vi "Example.vi"() -> ()   [LabVIEW 2015]
uses:
  <vilib>/Platform/TimedLoop/XDataNode/wakeup.ctl
  <vilib>/Platform/TimedLoop/XDataNode/XDNodeRunTimeDep.lvlib
  <vilib>/Platform/TimedLoop/XDataNode/nitl_modes.ctl
  <vilib>/Platform/TimedLoop/XDataNode/timing_clust.ctl
  <vilib>/Platform/TimedLoop/XDataNode/XDataNode.xnode
  <vilib>/NI/Engine Simulation Toolkit (EST)/APU/APU.lvlib
  <vilib>/rvi/DataTransferAndStorage/Container/XNode/niFpgaContainer.xnode
  <vilib>/rvi/interface/RandomDataEmulation/nirviRandomDataFpgaReadWriteTemplate.vi
  <vilib>/NI/Engine Simulation Toolkit (EST)/Directional Speed/Directional Speed.lvlib
  <vilib>/NI/Engine Simulation Toolkit (EST)/Digital Pattern Generation/Digital Pattern Generation.lvlib
  <vilib>/NI/Engine Simulation Toolkit (EST)/Analog Replay/Analog Replay.lvlib
  <vilib>/NI/FPGA Addon IP/Speciality IO/Speciality FPGA IO.lvlib
  <vilib>/NI/Engine Simulation Toolkit (EST)/Knock Sensor/Knock Sensor.lvlib
  <vilib>/NI/Engine Simulation Toolkit (EST)/ECU Event/Timing/ECU Event Timing.lvlib
  <vilib>/NI/Engine Simulation Toolkit (EST)/ECU Event/Timing/Measure Events (Non-40MHz).vi
  <vilib>/NI/Engine Simulation Toolkit (EST)/ECU Event/Timing/Capture Settings.ctl
  <vilib>/NI/Engine Simulation Toolkit (EST)/APU/Shared Settings.ctl
  <vilib>/NI/Engine Simulation Toolkit (EST)/Version Token.ctl
  <vilib>/NI/Engine Simulation Toolkit (EST)/Engine Simulation Toolkit.lvlib
  <vilib>/NI/Engine Simulation Toolkit (EST)/APU/Settings.ctl
  <vilib>/NI/Engine Simulation Toolkit (EST)/APU/Input.ctl
  <vilib>/NI/Engine Simulation Toolkit (EST)/APU/Output.ctl
  <vilib>/NI/Engine Simulation Toolkit (EST)/Directional Speed/Load Input.ctl
  <vilib>/NI/Engine Simulation Toolkit (EST)/Digital Pattern Generation/Load Input.ctl
  <vilib>/NI/Engine Simulation Toolkit (EST)/Analog Replay/Load Input.ctl
  <vilib>/NI/FPGA Addon IP/Speciality IO/Types/PWM.Measure.Analog.Settings.ctl
  <vilib>/NI/FPGA Addon IP/Speciality IO/Types/PWM.Measure.Analog.Measurement.ctl
  <vilib>/NI/Engine Simulation Toolkit (EST)/Knock Sensor/Cylinder Settings.ctl
  <vilib>/NI/Engine Simulation Toolkit (EST)/Knock Sensor/Cylinder Input.ctl
  <vilib>/NI/Engine Simulation Toolkit (EST)/Knock Sensor/Generate Settings.ctl
  <vilib>/NI/Engine Simulation Toolkit (EST)/Knock Sensor/Generate Input.ctl
  <vilib>/NI/FPGA Addon IP/Speciality IO/Types/Sine.Generate.Settings.ctl
  <vilib>/NI/Engine Simulation Toolkit (EST)/Analog Replay/Input.ctl
  <vilib>/NI/Engine Simulation Toolkit (EST)/Analog Replay/Settings.ctl
  <vilib>/NI/Engine Simulation Toolkit (EST)/Directional Speed/Input.ctl
  <vilib>/NI/Engine Simulation Toolkit (EST)/Directional Speed/Settings.ctl
  <vilib>/NI/Engine Simulation Toolkit (EST)/Digital Pattern Generation/Input.ctl
  <vilib>/NI/Engine Simulation Toolkit (EST)/Digital Pattern Generation/Settings.ctl
  <vilib>/NI/FPGA Addon IP/Speciality IO/Types/PWM.Generate.Digital.Settings.ctl
  <vilib>/NI/FPGA Addon IP/Speciality IO/Types/WSS.Generate.Digital.Settings.ctl
  <vilib>/NI/Engine Simulation Toolkit (EST)/ECU Event/Timing/Measure Settings.ctl
  <vilib>/NI/Engine Simulation Toolkit (EST)/ECU Event/Timing/Measure Output.ctl
  <vilib>/NI/Engine Simulation Toolkit (EST)/ECU Event/Timing/Capture Output.ctl
  <vilib>/NI/FPGA Addon IP/Speciality IO/Types/PWM.Measure.Digital.Settings.ctl
  <vilib>/NI/FPGA Addon IP/Speciality IO/Types/PWM.Measure.Digital.Measurement.ctl
panel:
  out "Switch State":bool
  out "Relay State":bool
  out "PWM IN 2.Measure":T1
  in  "PWM IN 2.Settings":T2={"ACTIVE EDGE"=TRUE, "TIMEOUT"=40000000}
  out "PWM IN 1.Measure":T1
  in  "PWM IN 1.Settings":T2={"ACTIVE EDGE"=TRUE, "TIMEOUT"=40000000}
  out "Key State":bool
  out "capture.Cyl Inj 3.Event 4":T3
  out "capture.Cyl Inj 3.Event 3":T3
  out "capture.Cyl Inj 3.Event 2":T3
  out "capture.Cyl Inj 3.Event 1":T3
  out "status.Cyl Inj 3":T4
  in  "settings.Cyl Inj 3":T5
  out "capture.Cyl Inj 2.Event 4":T3
  out "capture.Cyl Inj 2.Event 3":T3
  out "capture.Cyl Inj 2.Event 2":T3
  out "capture.Cyl Inj 2.Event 1":T3
  out "status.Cyl Inj 2":T4
  in  "settings.Cyl Inj 2":T5
  out "capture.Cyl Inj 1.Event 4":T3
  out "capture.Cyl Inj 1.Event 3":T3
  out "capture.Cyl Inj 1.Event 2":T3
  out "capture.Cyl Inj 1.Event 1":T3
  out "status.Cyl Inj 1":T4
  in  "settings.Cyl Inj 1":T5
  out "Test.Monitor":bool[](array[boolean])
  out "Mod5.Monitor":bool[](array[boolean])
  in  "Rear Driver WS.Settings":T6={"ACTIVE EDGE"=TRUE, "ACTIVE TICKS"=0, "INACTIVE TICKS"=0, "DATA"=0, "SENSOR TYPE"=0}
  in  "Read Passenger WS.Settings":T6={"ACTIVE EDGE"=TRUE, "ACTIVE TICKS"=0, "INACTIVE TICKS"=0, "DATA"=0, "SENSOR TYPE"=0}
  in  "Front Passenger WS.Settings":T6={"ACTIVE EDGE"=TRUE, "ACTIVE TICKS"=0, "INACTIVE TICKS"=0, "DATA"=0, "SENSOR TYPE"=0}
  in  "Front Driver WS.Settings":T6={"ACTIVE EDGE"=TRUE, "ACTIVE TICKS"=0, "INACTIVE TICKS"=0, "DATA"=0, "SENSOR TYPE"=0}
  out "Mod3.Monitor":bool[](array[boolean])
  in  "Switch":bool
  in  "PWM Out 2.Settings":T7={"ACTIVE EDGE"=TRUE, "ACTIVE TICKS"=0, "INACTIVE TICKS"=0}
  in  "PWM Out 1.Settings":T7={"ACTIVE EDGE"=TRUE, "ACTIVE TICKS"=0, "INACTIVE TICKS"=0}
  in  "Key":bool
  in  "input.Intake CAM 1":T8
  in  "settings.Intake CAM 1":T9
  in  "input.Exhaust CAM 1":T8
  in  "settings.Exhaust CAM 1":T9
  in  "input.Crank_Temp":T8
  in  "settings.Crank_Temp":T9
  in  "input.Crank":T10
  in  "settings.Crank":T11
  out "Mod4.Monitor":fxp<+/-,32,8>[](array[numeric])
  in  "input.VR Sensor4":T12
  in  "settings.VR Sensor4":T13
  in  "input.VR Sensor3":T12
  in  "settings.VR Sensor3":T13
  in  "input.VR Sensor2":T12
  in  "settings.VR Sensor2":T13
  in  "input.VR Sensor1":T12
  in  "settings.VR Sensor1":T13
  in  "Simple Knock 2.Settings":T14={"AMP"=0.0, "OFFSET"=0.0, "PERIODS/TICKS"=2.4999957531690598e-05}
  in  "Simple Knock 1.Settings":T14={"AMP"=0.0, "OFFSET"=0.0, "PERIODS/TICKS"=2.4999957531690598e-05}
  in  "Power Supply Setpoint":fxp<+/-,32,8> format="%#_27g"
  in  "input.Knock2":T15
  in  "settings.Knock2":T16
  in  "input.Knock2.Cylinder 6":T17={"probability compare"=65535, "high freq scaler"=0.0, "trigger position"=0}
  in  "settings.Knock2.Cylinder 6":T18
  in  "input.Knock2.Cylinder 5":T17={"probability compare"=65535, "high freq scaler"=0.0, "trigger position"=0}
  in  "settings.Knock2.Cylinder 5":T18
  in  "input.Knock2.Cylinder 4":T17={"probability compare"=65535, "high freq scaler"=0.0, "trigger position"=0}
  in  "settings.Knock2.Cylinder 4":T18
  in  "input.Knock2.Cylinder 3":T17={"probability compare"=65535, "high freq scaler"=0.0, "trigger position"=0}
  in  "settings.Knock2.Cylinder 3":T18
  in  "input.Knock2.Cylinder 2":T17={"probability compare"=65535, "high freq scaler"=0.0, "trigger position"=0}
  in  "settings.Knock2.Cylinder 2":T18
  in  "input.Knock2.Cylinder 1":T17={"probability compare"=65535, "high freq scaler"=0.0, "trigger position"=0}
  in  "settings.Knock2.Cylinder 1":T18
  in  "input.Knock1":T15
  in  "settings.Knock1":T16
  in  "input.Knock1.Cylinder 6":T17={"probability compare"=65535, "high freq scaler"=0.0, "trigger position"=0}
  in  "settings.Knock1.Cylinder 6":T18
  in  "input.Knock1.Cylinder 5":T17={"probability compare"=65535, "high freq scaler"=0.0, "trigger position"=0}
  in  "settings.Knock1.Cylinder 5":T18
  in  "input.Knock1.Cylinder 4":T17={"probability compare"=65535, "high freq scaler"=0.0, "trigger position"=0}
  in  "settings.Knock1.Cylinder 4":T18
  in  "input.Knock1.Cylinder 3":T17={"probability compare"=65535, "high freq scaler"=0.0, "trigger position"=0}
  in  "settings.Knock1.Cylinder 3":T18
  in  "input.Knock1.Cylinder 2":T17={"probability compare"=65535, "high freq scaler"=0.0, "trigger position"=0}
  in  "settings.Knock1.Cylinder 2":T18
  in  "input.Knock1.Cylinder 1":T17={"probability compare"=65535, "high freq scaler"=0.0, "trigger position"=0}
  in  "settings.Knock1.Cylinder 1":T18
  in  "Dyno Setpoint":fxp<+/-,32,8> format="%#_27g"
  out "Temp4":fxp<+/-,32,8> format="%#_27g"
  out "Temp3":fxp<+/-,32,8> format="%#_27g"
  out "Temp2":fxp<+/-,32,8> format="%#_27g"
  out "Temp1":fxp<+/-,32,8> format="%#_27g"
  out "Pressure2":fxp<+/-,32,8> format="%#_27g"
  out "Pressure1":fxp<+/-,32,8> format="%#_27g"
  out "Injector4.Measure":T19
  in  "Injector4.Settings":T20={"ACTIVE EDGE"=TRUE, "TIMEOUT"=40000000, "THRESHOLD"=50.0}
  out "Injector3.Measure":T19
  in  "Injector3.Settings":T20={"ACTIVE EDGE"=TRUE, "TIMEOUT"=40000000, "THRESHOLD"=50.0}
  out "Injector2.Measure":T19
  in  "Injector2.Settings":T20={"ACTIVE EDGE"=TRUE, "TIMEOUT"=40000000, "THRESHOLD"=50.0}
  out "Injector1.Measure":T19
  in  "Injector1.Settings":T20={"ACTIVE EDGE"=TRUE, "TIMEOUT"=40000000, "THRESHOLD"=50.0}
  out "Mod2.Monitor":fxp<+/-,24,5>[](array[numeric])
  in  "load input.VR Sensor4":T21={"Data"=[0, 0, 0, 0, 0, 0, 0, 0, 0, 0, 0, 0, 0, 0, 0, 0], "LoadOffset"=0, "Done"=FALSE}
  in  "load input.VR Sensor3":T21={"Data"=[0, 0, 0, 0, 0, 0, 0, 0, 0, 0, 0, 0, 0, 0, 0, 0], "LoadOffset"=0, "Done"=FALSE}
  in  "load input.VR Sensor2":T21={"Data"=[0, 0, 0, 0, 0, 0, 0, 0, 0, 0, 0, 0, 0, 0, 0, 0], "LoadOffset"=0, "Done"=FALSE}
  in  "load input.VR Sensor1":T21={"Data"=[0, 0, 0, 0, 0, 0, 0, 0, 0, 0, 0, 0, 0, 0, 0, 0], "LoadOffset"=0, "Done"=FALSE}
  in  "load input.Intake CAM 1":T22
  in  "load input.Exhaust CAM 1":T22
  in  "load input.Crank_Temp":T22
  in  "load input.Crank":T23
  in  "Analog Input Loop Timer (uSec)":u32
  out "output.apu 1":T24 caption="output"
  in  "input.apu 1":T25={"desired speed"=0.0, "reset"=TRUE} caption="input"
  in  "settings.apu 1":T26 caption="settings"
  in  "est.version":T27
  in  "shared settings.apu 1":T28 {"start" format="%#.15g"}
  in  "go.apu 1":bool
  in  "Digital Loop Timer (uSec)":u32
  in  "Analog Output Loop Timer (uSec)":u32
  in  "DMA.Enable":bool
  in  "DMA.MinimumSamples":u32 caption="DMA Loop Timer (uSec)"
  out "DMA.Timeout":bool
  in  "DMA.Timeout.Reset":bool
  in  "DMA Loop Timer (uSec)":u32
types:
  T1 = typedef "Speciality FPGA IO.lvlib/PWM.Measure.Digital.Measurement.ctl" = cluster{"ACTIVE TICKS":u32, "INACTIVE TICKS":u32, "ACQ TICKS":u32}
  T2 = typedef "Speciality FPGA IO.lvlib/PWM.Measure.Digital.Settings.ctl" = cluster{"ACTIVE EDGE":bool, "TIMEOUT":u32}
  T3 = typedef "Engine Simulation Toolkit.lvlib/ECU Event Timing.lvlib/Capture Output.ctl" = cluster{"Start":u16, "End":u16, "Duration (tics)":fxp<+,18,18>, "Event present":bool}
  T4 = typedef "Engine Simulation Toolkit.lvlib/ECU Event Timing.lvlib/Measure Output.ctl" = cluster{"stuck active":bool, "window all active":bool, "window orphan start":bool, "window orphan end":bool}
  T5 = typedef "Engine Simulation Toolkit.lvlib/ECU Event Timing.lvlib/Measure Settings.ctl" = cluster{"max":u16, "min":u16, "active high":bool, "wrap":bool}
  T6 = typedef "Speciality FPGA IO.lvlib/WSS.Generate.Digital.Settings.ctl" = cluster{"ACTIVE EDGE":bool, "ACTIVE TICKS":u32, "INACTIVE TICKS":u32, "DATA":u8, "SENSOR TYPE":u8}
  T7 = typedef "Speciality FPGA IO.lvlib/PWM.Generate.Digital.Settings.ctl" = cluster{"ACTIVE EDGE":bool, "ACTIVE TICKS":u32, "INACTIVE TICKS":u32}
  T8 = typedef "Engine Simulation Toolkit.lvlib/Digital Pattern Generation.lvlib/Settings.ctl" = cluster{"edge 1":u16, "edge 2":u16, "cycle angle":bool, "enabled":bool, "first falling":bool, "fault":bool, "fault wrap":bool, "fault value":bool, "fault count":fxp<+,4,4>, "use fault count":bool}
  T9 = typedef "Engine Simulation Toolkit.lvlib/Digital Pattern Generation.lvlib/Input.ctl" = cluster{"Offset":i16}
  T10 = typedef "Engine Simulation Toolkit.lvlib/Directional Speed.lvlib/Settings.ctl" = cluster{"Upper Value":u16, "Lower Value":u16, "Upper Index":fxp<+,10,10>, "Lower Index":fxp<+,10,10>, "Enabled":bool}
  T11 = typedef "Engine Simulation Toolkit.lvlib/Directional Speed.lvlib/Input.ctl" = cluster{"td (tics)":u16, "tf (tics)":u16, "tr (tics)":u16}
  T12 = typedef "Engine Simulation Toolkit.lvlib/Analog Replay.lvlib/Settings.ctl" = cluster{"ReverseNegate":bool, "CycleAngle":bool, "SpeedThreshold":fxp<+/-,23,2>, "AOBelowThreshold":i16}
  T13 = typedef "Engine Simulation Toolkit.lvlib/Analog Replay.lvlib/Input.ctl" = cluster{"Offset":i16, "VScaleSlope":fxp<+,18,6>, "VScaleIntercept":fxp<+/-,18,3>}
  T14 = typedef "Speciality FPGA IO.lvlib/Sine.Generate.Settings.ctl" = cluster{"AMP":fxp<+/-,32,8>, "OFFSET":fxp<+/-,32,8>, "PERIODS/TICKS":fxp<+,32,0>}
  T15 = typedef "Engine Simulation Toolkit.lvlib/Knock Sensor.lvlib/Generate Input.ctl" = cluster{"low freq scaler":fxp<+,10,0>}
  T16 = typedef "Engine Simulation Toolkit.lvlib/Knock Sensor.lvlib/Generate Settings.ctl" = cluster{"low freq (periods/tick)":fxp<+,32,0>, "high freq (periods/tick)":fxp<+,32,0>, "duration (1.25MHz tics)":fxp<+,18,18>, "low freq speed slope":fxp<+,16,-3>, "low freq speed intercept":fxp<+,10,-10>, "low freq by speed":bool}
  T17 = typedef "Engine Simulation Toolkit.lvlib/Knock Sensor.lvlib/Cylinder Input.ctl" = cluster{"probability compare":u16, "high freq scaler":fxp<+,10,0>, "trigger position":u16}
  T18 = typedef "Engine Simulation Toolkit.lvlib/Knock Sensor.lvlib/Cylinder Settings.ctl" = cluster{"seed":u16, "reset":bool}
  T19 = typedef "Speciality FPGA IO.lvlib/PWM.Measure.Analog.Measurement.ctl" = cluster{"ACTIVE TICKS":u32, "INACTIVE TICKS":u32, "ACQ TICKS":u32, "ACTIVE VOLTAGE":fxp<+/-,32,8>, "INACTIVE VOLTAGE":fxp<+/-,32,8>}
  T20 = typedef "Speciality FPGA IO.lvlib/PWM.Measure.Analog.Settings.ctl" = cluster{"ACTIVE EDGE":bool, "TIMEOUT":u32, "THRESHOLD":fxp<+/-,32,8>}
  T21 = typedef "Engine Simulation Toolkit.lvlib/Analog Replay.lvlib/Load Input.ctl" = cluster{"Data":i16[], "LoadOffset":u16, "Done":bool}
  T22 = typedef "Engine Simulation Toolkit.lvlib/Digital Pattern Generation.lvlib/Load Input.ctl" = cluster{"address":fxp<+,11,11>, "done":bool, "angle":u16}
  T23 = typedef "Engine Simulation Toolkit.lvlib/Directional Speed.lvlib/Load Input.ctl" = cluster{"address":fxp<+,10,10>, "done":bool, "angle":u16}
  T24 = typedef "Engine Simulation Toolkit.lvlib/APU.lvlib/Output.ctl" = cluster{"crank":u16, "cycle":u16, "actual speed":fxp<+/-,23,2>}
  T25 = typedef "Engine Simulation Toolkit.lvlib/APU.lvlib/Input.ctl" = cluster{"desired speed":fxp<+/-,23,2>, "reset":bool}
  T26 = typedef "Engine Simulation Toolkit.lvlib/APU.lvlib/Settings.ctl" = cluster{"acceleration":fxp<+,18,-20>, "enable accel":bool}
  T27 = typedef "Engine Simulation Toolkit.lvlib/Version Token.ctl" = cluster{"1.3.0":bool}
  T28 = typedef "Engine Simulation Toolkit.lvlib/APU.lvlib/Shared Settings.ctl" = cluster{"start":fxp<+,17,17>, "stuck limit":fxp<+,18,18>}
  T29 = typedef "XDNodeRunTimeDep.lvlib/timing_clust.ctl" = cluster{"Expected End [f-1]":u64, "Actual End [f-1]":u64, "Finished Late? [f-1]":bool, "Expected End [i-1]":u64, "Actual End [i-1]":u64, "Finished Late? [i-1]":bool, "Expected Start [i]":u64, "Actual Start [i]":u64, "Expected Start [f]":u64, "Actual Start [f]":u64, "Source Name":string, "Structure Name":string, "Period":i64, "Deadline":i64, "Offset":i64, "Start":i64, "Priority":i32, "Timeout":i32, "Mode":T30, "Wakeup Reason":T31, "Error":errorcluster, "Source Type":string, "Secondary Source Type":string, "Global End Time":u64, "Global Start Time":u64, "Frame Duration":u64, "Iteration Duration":u64, "Assigned CPU":i32, "I/O Scan Engine Mode":u32}
  T30 = typedef "XDNodeRunTimeDep.lvlib/nitl_modes.ctl" = enum32{"No Change", "Process missed periods, maintain original phase", "Discard missed periods, maintain original phase", "Process missed periods, ignore original phase", "Discard missed periods, ignore original phase"}
  T31 = typedef "XDNodeRunTimeDep.lvlib/wakeup.ctl" = enum32{"Normal", "Aborted", "Asynchronous wakeup", "Timing source error", "Timed loop error", "Timeout"}
  T32 = typedef "Engine Simulation Toolkit.lvlib/ECU Event Timing.lvlib/Capture Settings.ctl" = u8
  T33 = cluster{"DI 0":refnum<k21>, "DI 1":refnum<k21>, "DI 2":refnum<k21>, "DI 3":refnum<k21>, "DI 4":refnum<k21>, "DI 5":refnum<k21>, "DI 6":refnum<k21>, "DI 7":refnum<k21>}
  T34 = cluster{"DO 0":refnum<k21>, "DO 1":refnum<k21>, "DO 2":refnum<k21>, "DO 3":refnum<k21>, "DO 4":refnum<k21>, "DO 5":refnum<k21>, "DO 6":refnum<k21>, "DO 7":refnum<k21>}
  T35 = cluster{"AO 0":refnum<k21>, "AO 1":refnum<k21>, "AO 2":refnum<k21>, "AO 3":refnum<k21>, "AO 4":refnum<k21>, "AO 5":refnum<k21>, "AO 6":refnum<k21>, "AO 7":refnum<k21>, "AO 8":refnum<k21>, "AO 9":refnum<k21>, "AO 10":refnum<k21>, "AO 11":refnum<k21>, "AO 12":refnum<k21>, "AO 13":refnum<k21>, "AO 14":refnum<k21>, "AO 15":refnum<k21>}
  T36 = cluster{"AI 0":refnum<k21>, "AI 1":refnum<k21>, "AI 2":refnum<k21>, "AI 3":refnum<k21>, "AI 4":refnum<k21>, "AI 5":refnum<k21>, "AI 6":refnum<k21>, "AI 7":refnum<k21>, "AI 8":refnum<k21>, "AI 9":refnum<k21>, "AI 10":refnum<k21>, "AI 11":refnum<k21>, "AI 12":refnum<k21>, "AI 13":refnum<k21>, "AI 14":refnum<k21>, "AI 15":refnum<k21>}
  T37 = typedef "Engine Simulation Toolkit.lvlib/APU.lvlib/Register Bus.ctl" = cluster{"Speed":refnum<k21>, "Crank Angle":refnum<k21>, "Cycle Angle":refnum<k21>, "Crank Count":refnum<k21>, "Cycle Count":refnum<k21>, "1.25 MHz Counter":refnum<k21>, "Crank Rollover":refnum<k21>, "Cycle Rollover":refnum<k21>, "shared settings":T28}
  T38 = typedef "Engine Simulation Toolkit.lvlib/Directional Speed.lvlib/Load Data.ctl" = cluster{"max address":fxp<+,10,10>, "Memory":refnum<k21>}
  T39 = typedef "Engine Simulation Toolkit.lvlib/Digital Pattern Generation.lvlib/Load Data.ctl" = cluster{"max address":fxp<+,11,11>, "memory":refnum<k21>}
  T40 = typedef "Engine Simulation Toolkit.lvlib/Knock Sensor.lvlib/Triggered Cylinder Data.ctl" = cluster{"trigger knock":bool, "high freq scaler":fxp<+,10,0>}
  T41 = typedef "Engine Simulation Toolkit.lvlib/ECU Event Timing.lvlib/Measured Data.ctl" = cluster{"start":u16, "end":u16, "duration (tics)":fxp<+,18,18>, "window end":bool, "window begin":bool, "pulse end":bool, "pulse #":u8}
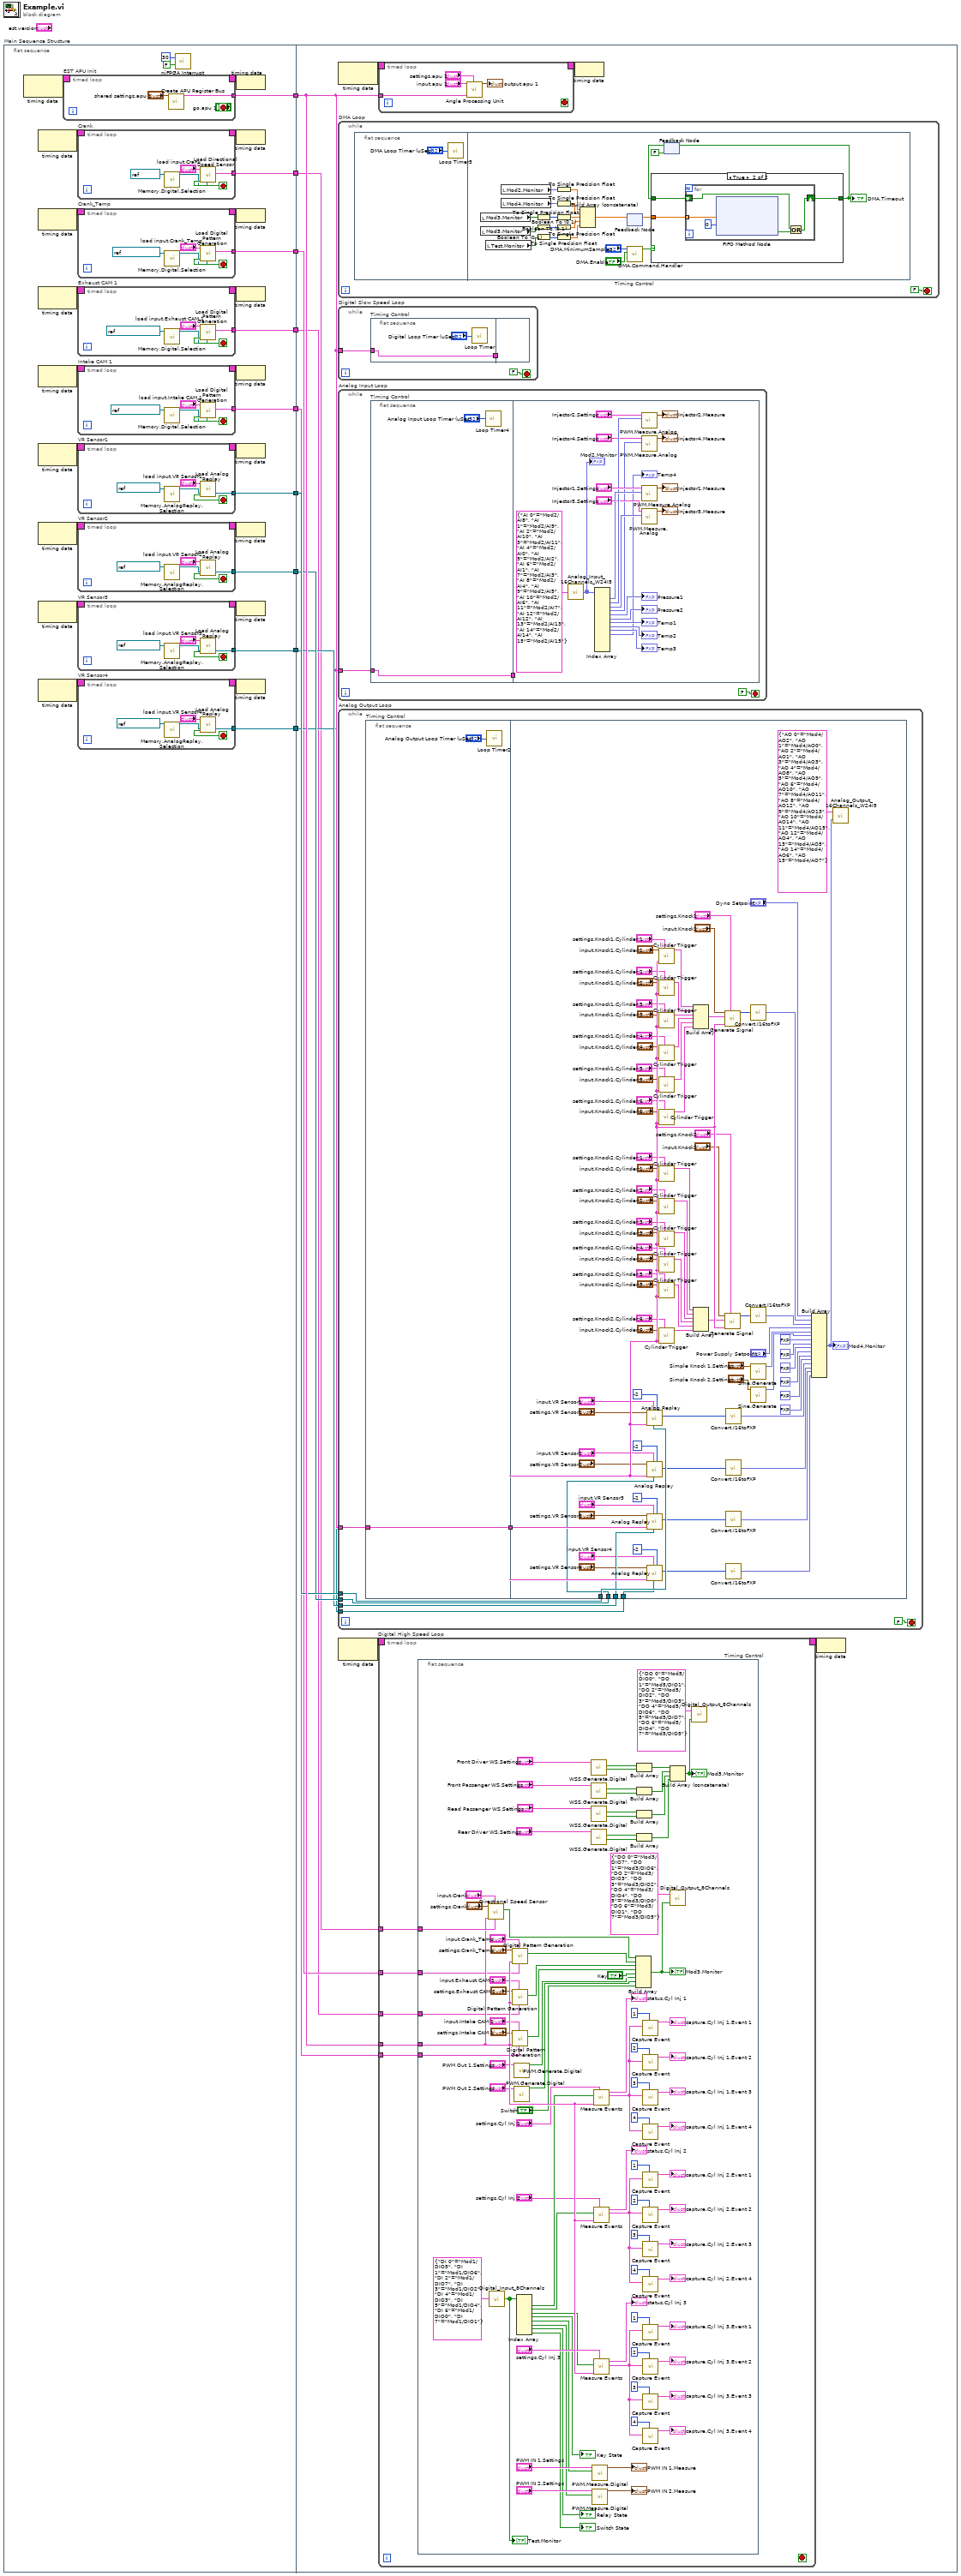
[diagram p0: block diagram]
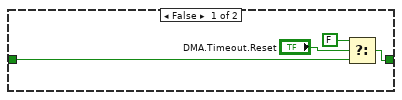
[diagram p2: hidden frame]
diagram:
  n1 = flat-sequence "Main Sequence Structure" {
    tunnel: [w34] -> w9
    tunnel: [w17] -> w8
    tunnel: [w16] -> w7
    tunnel: [w15] -> w6
    tunnel: [w14] -> w5
    tunnel: [w13] -> w4
    tunnel: [w12] -> w3
    tunnel: [w11] -> w2
    tunnel: [w10] -> w1
    tunnel: w9 -> [w122]
    tunnel: w8 -> [w121]
    tunnel: w7 -> [w120]
    tunnel: w6 -> [w119]
    tunnel: w5 -> [w118]
    tunnel: w4 -> [w117]
    tunnel: w3 -> [w116]
    tunnel: w2 -> [w115]
    tunnel: w1 -> [w114]
    frame #0 {
      n2 = node-c288() -> (w36:T29)  [unwired: 1 in]
      n3 = node-c288() -> (w33:T29)  [unwired: 1 in]
      n4 = node-c288() -> (w31:T29)  [unwired: 1 in]
      n5 = node-c288() -> (w29:T29)  [unwired: 1 in]
      n6 = node-c288() -> (w27:T29)  [unwired: 1 in]
      n7 = node-c288() -> (w25:T29)  [unwired: 1 in]
      n8 = node-c288() -> (w23:T29)  [unwired: 1 in]
      n9 = node-c288() -> (w21:T29)  [unwired: 1 in]
      n10 = node-c288() -> (w19:T29)  [unwired: 1 in]
      n11 = timed-loop "EST APU Init" {
        timing: w36 -> [_]
        timing-out: [_] -> w35
        tunnel: [w107] -> w34
        stop <- "go.apu 1" stop-if-true
        n12 = call <vilib>:"Create APU Register Bus.vi"("shared settings.<user name>"="shared settings.apu 1") -> ("register bus"=w107:T37)  [unwired: 10 in]
      }
      n13 = timed-loop "Crank" {
        timing: w33 -> [_]
        timing-out: [_] -> w32
        tunnel: [w98] -> w13
        stop <- w101 stop-if-true
        n14 = call "Memory.Digital.Selection.vi"("memory"=refnum<k21> "Crank") -> ("memory"=w99:refnum<k21>)  [unwired: 10 in]
        n15 = call <vilib>:"Load Directional Speed Sensor.vi"("Memory In"=w99, "load input.<user name>"="load input.Crank") -> ("done"=w101:bool, "load data"=w98:T38)  [unwired: 8 in]
      }
      n16 = timed-loop "Crank_Temp" {
        timing: w31 -> [_]
        timing-out: [_] -> w30
        tunnel: [w89] -> w12
        stop <- w92 stop-if-true
        n17 = call "Memory.Digital.Selection.vi"("memory"=refnum<k21> "Crank_Temp") -> ("memory"=w90:refnum<k21>)  [unwired: 10 in]
        n18 = call <vilib>:"Load Digital Pattern Generation.vi"("memory"=w90, "load input.<user name>"="load input.Crank_Temp") -> ("done"=w92:bool, "load data"=w89:T39)  [unwired: 8 in]
      }
      n19 = timed-loop "Exhaust CAM 1" {
        timing: w29 -> [_]
        timing-out: [_] -> w28
        tunnel: [w80] -> w11
        stop <- w83 stop-if-true
        n20 = call "Memory.Digital.Selection.vi"("memory"=refnum<k21> "Exhaust CAM 1") -> ("memory"=w81:refnum<k21>)  [unwired: 10 in]
        n21 = call <vilib>:"Load Digital Pattern Generation.vi"("memory"=w81, "load input.<user name>"="load input.Exhaust CAM 1") -> ("done"=w83:bool, "load data"=w80:T39)  [unwired: 8 in]
      }
      n22 = timed-loop "Intake CAM 1" {
        timing: w27 -> [_]
        timing-out: [_] -> w26
        tunnel: [w71] -> w10
        stop <- w74 stop-if-true
        n23 = call "Memory.Digital.Selection.vi"("memory"=refnum<k21> "Intake CAM 1") -> ("memory"=w72:refnum<k21>)  [unwired: 10 in]
        n24 = call <vilib>:"Load Digital Pattern Generation.vi"("memory"=w72, "load input.<user name>"="load input.Intake CAM 1") -> ("done"=w74:bool, "load data"=w71:T39)  [unwired: 8 in]
      }
      n25 = timed-loop "VR Sensor1" {
        timing: w25 -> [_]
        timing-out: [_] -> w24
        tunnel: [w63] -> w17
        stop <- w65 stop-if-true
        n26 = call "Memory.AnalogReplay.Selection.vi"("memory"=refnum<k21> "VR Sensor1") -> ("memory"=w63:refnum<k21>)  [unwired: 10 in]
        n27 = call <vilib>:"Load Analog Replay.vi"("memory"=w63, "load input.<user name>"="load input.VR Sensor1") -> ("done"=w65:bool)  [unwired: 9 in]
      }
      n28 = timed-loop "VR Sensor2" {
        timing: w23 -> [_]
        timing-out: [_] -> w22
        tunnel: [w55] -> w16
        stop <- w57 stop-if-true
        n29 = call "Memory.AnalogReplay.Selection.vi"("memory"=refnum<k21> "VR Sensor2") -> ("memory"=w55:refnum<k21>)  [unwired: 10 in]
        n30 = call <vilib>:"Load Analog Replay.vi"("memory"=w55, "load input.<user name>"="load input.VR Sensor2") -> ("done"=w57:bool)  [unwired: 9 in]
      }
      n31 = timed-loop "VR Sensor3" {
        timing: w21 -> [_]
        timing-out: [_] -> w20
        tunnel: [w47] -> w15
        stop <- w49 stop-if-true
        n32 = call "Memory.AnalogReplay.Selection.vi"("memory"=refnum<k21> "VR Sensor3") -> ("memory"=w47:refnum<k21>)  [unwired: 10 in]
        n33 = call <vilib>:"Load Analog Replay.vi"("memory"=w47, "load input.<user name>"="load input.VR Sensor3") -> ("done"=w49:bool)  [unwired: 9 in]
      }
      n34 = timed-loop "VR Sensor4" {
        timing: w19 -> [_]
        timing-out: [_] -> w18
        tunnel: [w39] -> w14
        stop <- w41 stop-if-true
        n35 = call "Memory.AnalogReplay.Selection.vi"("memory"=refnum<k21> "VR Sensor4") -> ("memory"=w39:refnum<k21>)  [unwired: 10 in]
        n36 = call <vilib>:"Load Analog Replay.vi"("memory"=w39, "load input.<user name>"="load input.VR Sensor4") -> ("done"=w41:bool)  [unwired: 9 in]
      }
      n37 = call <vilib>:"niFPGA Interrupt.vi"("Wait Until Cleared (F)"=FALSE, "IRQ Number (0)"=u8 30) -> ()  [unwired: 1 in]
      n38 = node-c288(w35) -> ()
      n39 = node-c288(w32) -> ()
      n40 = node-c288(w30) -> ()
      n41 = node-c288(w28) -> ()
      n42 = node-c288(w26) -> ()
      n43 = node-c288(w24) -> ()
      n44 = node-c288(w22) -> ()
      n45 = node-c288(w20) -> ()
      n46 = node-c288(w18) -> ()
    }
    frame #1 {
      # "FPGA Addon Code"
      n47 = node-c288 ("Input Node")() -> (w124:T29)  [unwired: 1 in]
      n48 = while "DMA Loop" {
        stop <- FALSE stop-if-true
        n49 = flat-sequence "Timing Control" {
          frame #0 {
            n50 = call "Loop Timer3"("Count(uSec)"="DMA Loop Timer (uSec)") -> ()  [unwired: 1 out]
          }
          frame #1 {
            n51 = local read "Mod3.Monitor"() -> (w246:bool[])
            n52 = local read "Mod5.Monitor"() -> (w244:bool[])
            n53 = local read "Test.Monitor"() -> (w242:bool[])
            n54 = local read "Mod2.Monitor"() -> (w248:fxp<+/-,24,5>[])
            n55 = local read "Mod4.Monitor"() -> (w247:fxp<+/-,32,8>[])
            n56 = Boolean To (0,1)(Boolean=w246) -> (0, 1=w245:i16[])
            n57 = Boolean To (0,1)(Boolean=w244) -> (0, 1=w243:i16[])
            n58 = Boolean To (0,1)(Boolean=w242) -> (0, 1=w241:i16[])
            n59 = To Single Precision Float(number=w248) -> (single precision float=w240:sgl[])
            n60 = To Single Precision Float(number=w247) -> (single precision float=w239:sgl[])
            n61 = To Single Precision Float(number=w245) -> (single precision float=w238:sgl[])
            n62 = To Single Precision Float(number=w243) -> (single precision float=w237:sgl[])
            n63 = To Single Precision Float(number=w241) -> (single precision float=w236:sgl[])
            n64 = Build Array (concatenate) "Build Array"(w240, w239, w238, w237, w236) -> (w254:sgl[])
            n65 = feedback #1() -> (w253:sgl[])  [unwired: 1 in]
            n66 = feedback-in #1(w254) -> ()
            n67 = call "DMA.Command.Handler.vi"("DMA.Enable"="DMA.Enable", "DMA.MinimumSamples"="DMA.MinimumSamples") -> ("Transfer"=w250:bool)  [unwired: 9 in]
            n68 = feedback #2(FALSE ("t")) -> (w249:bool)
            n69 = case shown="True" w250 {
              tunnel: w253 -> [_ w263]
              tunnel: w249 -> [w258 w262]
              tunnel: [w257 w261] -> w252
              frame False {
                n70 = Select(t=FALSE, s="DMA.Timeout.Reset", f=w258) -> (s? t:f=w257:bool)
              }
              frame True {
                n71 = for {
                  shift-right: [w266] -> w261
                  shift-left: w262 -> [w265]
                  tunnel: w263 -> [w264] mode=indexing
                  n72 = xnode ("FIFO Method Node")("Element"=w264, "Timeout"=0) -> ("Timed Out?"=w267:bool)  [unwired: 1 in, 1 out]
                  n73 = Or(x=w265, y=w267) -> (x .or. y?=w266:bool)
                }
              }
            }
            "DMA.Timeout" <- w252
            n74 = feedback-in #2(w252) -> ()
          }
        }
      }
      n75 = while "Digital Slow Speed Loop" {
        tunnel: w122 -> [w389]
        stop <- FALSE stop-if-true
        n76 = flat-sequence "Timing Control" {
          tunnel: w389 -> [w391]
          tunnel: [w391] -> w388
          tunnel: w388 -> [_]
          frame #0 {
            n77 = call "Loop Timer"("Count(uSec)"="Digital Loop Timer (uSec)") -> ()  [unwired: 1 out]
          }
          frame #1 {
          }
        }
      }
      n78 = while "Analog Input Loop" {
        tunnel: w122 -> [w364]
        stop <- FALSE stop-if-true
        n79 = flat-sequence "Timing Control" {
          tunnel: w364 -> [w366]
          tunnel: [w366] -> w363
          tunnel: w363 -> [_]
          frame #0 {
            n80 = call "Loop Timer4"("Count(uSec)"="Analog Input Loop Timer (uSec)") -> ()  [unwired: 1 out]
          }
          frame #1 {
            n81 = call "Analog_Input_16Channels_W24I5.vi"("IO"=T36 {"AI 0"="Mod2/AI8", "AI 1"="Mod2/AI9", "AI 2"="Mod2/AI10", "AI 3"="Mod2/AI11", "AI 4"="Mod2/AI0", "AI 5"="Mod2/AI2", "AI 6"="Mod2/AI1", "AI 7"="Mod2/AI3", "AI 8"="Mod2/AI4", "AI 9"="Mod2/AI5", "AI 10"="Mod2/AI6", "AI 11"="Mod2/AI7", "AI 12"="Mod2/AI12", "AI 13"="Mod2/AI13", "AI 14"="Mod2/AI14", "AI 15"="Mod2/AI15"}) -> ("Values"=w386:fxp<+/-,24,5>[])
            "Mod2.Monitor" <- w386
            n82 = Index Array(array=w386) -> (element #1=w384:fxp<+/-,24,5>, element #2=w381:fxp<+/-,24,5>, element #3=w378:fxp<+/-,24,5>, element #4=w375:fxp<+/-,24,5>, element #5=→"Pressure1":fxp<+/-,24,5>, element #6=→"Pressure2":fxp<+/-,24,5>, element #7=→"Temp1":fxp<+/-,24,5>, element #8=→"Temp2":fxp<+/-,24,5>, element #9=→"Temp3":fxp<+/-,24,5>, element #10=→"Temp4":fxp<+/-,24,5>)  [unwired: 14 in, 4 out]
            n83 = call <vilib>:"PWM.Measure.Analog.vi"("PWM"=w381, "Settings"="Injector2.Settings") -> ("Measurement"=→"Injector2.Measure":T19)  [unwired: 8 in, 1 out]
            n84 = call <vilib>:"PWM.Measure.Analog.vi"("PWM"=w375, "Settings"="Injector4.Settings") -> ("Measurement"=→"Injector4.Measure":T19)  [unwired: 8 in, 1 out]
            n85 = call <vilib>:"PWM.Measure.Analog.vi"("PWM"=w384, "Settings"="Injector1.Settings") -> ("Measurement"=→"Injector1.Measure":T19)  [unwired: 8 in, 1 out]
            n86 = call <vilib>:"PWM.Measure.Analog.vi"("PWM"=w378, "Settings"="Injector3.Settings") -> ("Measurement"=→"Injector3.Measure":T19)  [unwired: 8 in, 1 out]
          }
        }
      }
      n87 = while "Analog Output Loop" {
        tunnel: w122 -> [w274]
        tunnel: w121 -> [w272]
        tunnel: w120 -> [w271]
        tunnel: w119 -> [w270]
        tunnel: w118 -> [w269]
        stop <- FALSE stop-if-true
        n88 = flat-sequence "Timing Control" {
          tunnel: w274 -> [w276]
          tunnel: [w276] -> w273
          tunnel: w273 -> [w360]
          tunnel: w272 -> [w312]
          tunnel: w271 -> [w307]
          tunnel: w270 -> [w302]
          tunnel: w269 -> [w297]
          frame #0 {
            n89 = call "Loop Timer2"("Count(uSec)"="Analog Output Loop Timer (uSec)") -> ()  [unwired: 1 out]
          }
          frame #1 {
            n90 = call <vilib>:"Analog Replay.vi"("shift"=i8 -2, "memory"=w312, "settings.<user name>"="input.VR Sensor1", "register bus"=w360, "input.<user name>"="settings.VR Sensor1") -> ("analog value"=w311:i16)  [unwired: 6 in]
            n91 = call <vilib>:"Analog Replay.vi"("shift"=i8 -2, "memory"=w307, "settings.<user name>"="input.VR Sensor2", "register bus"=w360, "input.<user name>"="settings.VR Sensor2") -> ("analog value"=w306:i16)  [unwired: 6 in]
            n92 = call <vilib>:"Analog Replay.vi"("shift"=i8 -2, "memory"=w302, "settings.<user name>"="input.VR Sensor3", "register bus"=w360, "input.<user name>"="settings.VR Sensor3") -> ("analog value"=w301:i16)  [unwired: 6 in]
            n93 = call <vilib>:"Analog Replay.vi"("shift"=i8 -2, "memory"=w297, "settings.<user name>"="input.VR Sensor4", "register bus"=w360, "input.<user name>"="settings.VR Sensor4") -> ("analog value"=w296:i16)  [unwired: 6 in]
            n94 = call <vilib>:"Cylinder Trigger.vi"("settings.<user name>"="settings.Knock1.Cylinder 1", "register bus"=w360, "input.<user name>"="input.Knock1.Cylinder 1") -> ("triggered knock data"=w359:T40)  [unwired: 8 in]
            n95 = call <vilib>:"Cylinder Trigger.vi"("settings.<user name>"="settings.Knock1.Cylinder 2", "register bus"=w360, "input.<user name>"="input.Knock1.Cylinder 2") -> ("triggered knock data"=w356:T40)  [unwired: 8 in]
            n96 = call <vilib>:"Cylinder Trigger.vi"("settings.<user name>"="settings.Knock1.Cylinder 3", "register bus"=w360, "input.<user name>"="input.Knock1.Cylinder 3") -> ("triggered knock data"=w353:T40)  [unwired: 8 in]
            n97 = call <vilib>:"Cylinder Trigger.vi"("settings.<user name>"="settings.Knock1.Cylinder 4", "register bus"=w360, "input.<user name>"="input.Knock1.Cylinder 4") -> ("triggered knock data"=w350:T40)  [unwired: 8 in]
            n98 = call <vilib>:"Cylinder Trigger.vi"("settings.<user name>"="settings.Knock1.Cylinder 5", "register bus"=w360, "input.<user name>"="input.Knock1.Cylinder 5") -> ("triggered knock data"=w347:T40)  [unwired: 8 in]
            n99 = call <vilib>:"Cylinder Trigger.vi"("settings.<user name>"="settings.Knock1.Cylinder 6", "register bus"=w360, "input.<user name>"="input.Knock1.Cylinder 6") -> ("triggered knock data"=w344:T40)  [unwired: 8 in]
            n100 = call <vilib>:"Cylinder Trigger.vi"("settings.<user name>"="settings.Knock2.Cylinder 1", "register bus"=w360, "input.<user name>"="input.Knock2.Cylinder 1") -> ("triggered knock data"=w337:T40)  [unwired: 8 in]
            n101 = call <vilib>:"Cylinder Trigger.vi"("settings.<user name>"="settings.Knock2.Cylinder 2", "register bus"=w360, "input.<user name>"="input.Knock2.Cylinder 2") -> ("triggered knock data"=w334:T40)  [unwired: 8 in]
            n102 = call <vilib>:"Cylinder Trigger.vi"("settings.<user name>"="settings.Knock2.Cylinder 3", "register bus"=w360, "input.<user name>"="input.Knock2.Cylinder 3") -> ("triggered knock data"=w331:T40)  [unwired: 8 in]
            n103 = call <vilib>:"Cylinder Trigger.vi"("settings.<user name>"="settings.Knock2.Cylinder 4", "register bus"=w360, "input.<user name>"="input.Knock2.Cylinder 4") -> ("triggered knock data"=w328:T40)  [unwired: 8 in]
            n104 = call <vilib>:"Cylinder Trigger.vi"("settings.<user name>"="settings.Knock2.Cylinder 5", "register bus"=w360, "input.<user name>"="input.Knock2.Cylinder 5") -> ("triggered knock data"=w325:T40)  [unwired: 8 in]
            n105 = call <vilib>:"Cylinder Trigger.vi"("settings.<user name>"="settings.Knock2.Cylinder 6", "register bus"=w360, "input.<user name>"="input.Knock2.Cylinder 6") -> ("triggered knock data"=w322:T40)  [unwired: 8 in]
            n106 = Build Array(w359, w356, w353, w350, w347, w344) -> (w341:T40[])
            n107 = Build Array(w337, w334, w331, w328, w325, w322) -> (w319:T40[])
            n108 = call <vilib>:"Generate Signal.vi"("settings.<user name>"="settings.Knock1", "register bus"=w360, "triggered knock data"=w341, "input.<user name>"="input.Knock1") -> ("knock signal"=w340:i16)  [unwired: 7 in]
            n109 = call <vilib>:"Generate Signal.vi"("settings.<user name>"="settings.Knock2", "register bus"=w360, "triggered knock data"=w319, "input.<user name>"="input.Knock2") -> ("knock signal"=w318:i16)  [unwired: 7 in]
            n110 = call "Convert.I16toFXP.vi"("16bit integer"=w311) -> ("x*y"=w283:fxp<+/-,20,5>)  [unwired: 4 in]
            n111 = call "Convert.I16toFXP.vi"("16bit integer"=w306) -> ("x*y"=w282:fxp<+/-,20,5>)  [unwired: 4 in]
            n112 = call "Convert.I16toFXP.vi"("16bit integer"=w301) -> ("x*y"=w281:fxp<+/-,20,5>)  [unwired: 4 in]
            n113 = call "Convert.I16toFXP.vi"("16bit integer"=w296) -> ("x*y"=w280:fxp<+/-,20,5>)  [unwired: 4 in]
            n114 = call "Convert.I16toFXP.vi"("16bit integer"=w340) -> ("x*y"=w294:fxp<+/-,20,5>)  [unwired: 4 in]
            n115 = call "Convert.I16toFXP.vi"("16bit integer"=w318) -> ("x*y"=w293:fxp<+/-,20,5>)  [unwired: 4 in]
            n116 = call <vilib>:"Sine.Generate.vi"("Settings"="Simple Knock 1.Settings") -> ("Output"=w291:fxp<+/-,32,8>)  [unwired: 10 in]
            n117 = call <vilib>:"Sine.Generate.vi"("Settings"="Simple Knock 2.Settings") -> ("Output"=w290:fxp<+/-,32,8>)  [unwired: 10 in]
            n118 = Build Array("Dyno Setpoint", w294, w293, "Power Supply Setpoint", w291, w290, fxp<+/-,32,8> 0.0, fxp<+/-,32,8> 0.0, fxp<+/-,32,8> 0.0, fxp<+/-,32,8> 0.0, fxp<+/-,32,8> 0.0, fxp<+/-,32,8> 0.0, w283, w282, w281, w280) -> (w278:fxp<+/-,32,8>[])
            "Mod4.Monitor" <- w278
            n119 = call "Analog_Output_16Channels_W24I5.vi"("Values"=w278, "IO"=T35 {"AO 0"="Mod4/AO2", "AO 1"="Mod4/AO0", "AO 2"="Mod4/AO1", "AO 3"="Mod4/AO3", "AO 4"="Mod4/AO8", "AO 5"="Mod4/AO9", "AO 6"="Mod4/AO10", "AO 7"="Mod4/AO11", "AO 8"="Mod4/AO12", "AO 9"="Mod4/AO13", "AO 10"="Mod4/AO14", "AO 11"="Mod4/AO15", "AO 12"="Mod4/AO4", "AO 13"="Mod4/AO5", "AO 14"="Mod4/AO6", "AO 15"="Mod4/AO7"}) -> ()  [unwired: 1 in]
          }
        }
      }
      n120 = node-c288() -> (w126:T29)  [unwired: 1 in]
      n121 = timed-loop "Timed Loop" {
        timing: w124 -> [_]
        timing-out: [_] -> w123
        tunnel: w122 -> [w127]
        stop <- _ stop-if-true
        n122 = call <vilib>:"Angle Processing Unit.vi"("settings.<user name>"="settings.apu 1", "register bus"=w127, "input.<user name>"="input.apu 1") -> ("output.<user name>"=→"output.apu 1":T24)  [unwired: 8 in]
      }
      n123 = timed-loop "Digital High Speed Loop" {
        timing: w126 -> [_]
        timing-out: [_] -> w125
        tunnel: w122 -> [w139]
        tunnel: w117 -> [w138]
        tunnel: w116 -> [w137]
        tunnel: w115 -> [w136]
        tunnel: w114 -> [w135]
        stop <- _ stop-if-true
        n124 = flat-sequence "Timing Control" {
          tunnel: w139 -> [w226]
          tunnel: w138 -> [w227]
          tunnel: w137 -> [w223]
          tunnel: w136 -> [w220]
          tunnel: w135 -> [w217]
          frame #0 {
            n125 = call <vilib>:"Directional Speed Sensor.vi"("load data"=w227, "settings.<user name>"="input.Crank", "register bus"=w226, "input.<user name>"="settings.Crank") -> ("digial output"=w214:bool)  [unwired: 7 in]
            n126 = call "Digital_Input_8Channels.vi"("IO"=T33 {"DI 0"="Mod1/DIO5", "DI 1"="Mod1/DIO6", "DI 2"="Mod1/DIO7", "DI 3"="Mod1/DIO2", "DI 4"="Mod1/DIO3", "DI 5"="Mod1/DIO4", "DI 6"="Mod1/DIO0", "DI 7"="Mod1/DIO1"}) -> ("States"=w185:bool[])
            "Test.Monitor" <- w185
            n127 = call <vilib>:"Digital Pattern Generation.vi"("load data"=w223, "settings.<user name>"="input.Crank_Temp", "register bus"=w226, "input.<user name>"="settings.Crank_Temp") -> ("digial output"=w213:bool)  [unwired: 7 in]
            n128 = call <vilib>:"Digital Pattern Generation.vi"("load data"=w220, "settings.<user name>"="input.Exhaust CAM 1", "register bus"=w226, "input.<user name>"="settings.Exhaust CAM 1") -> ("digial output"=w212:bool)  [unwired: 7 in]
            n129 = call <vilib>:"Digital Pattern Generation.vi"("load data"=w217, "settings.<user name>"="input.Intake CAM 1", "register bus"=w226, "input.<user name>"="settings.Intake CAM 1") -> ("digial output"=w211:bool)  [unwired: 7 in]
            n130 = call <vilib>:"PWM.Generate.Digital.vi"("Settings"="PWM Out 1.Settings") -> ("Output"=w209:bool)  [unwired: 10 in]
            n131 = call <vilib>:"PWM.Generate.Digital.vi"("Settings"="PWM Out 2.Settings") -> ("Output"=w208:bool)  [unwired: 10 in]
            n132 = Index Array(array=w185) -> (element #1=w183:bool, element #2=w171:bool, element #3=w159:bool, element #4=→"Key State":bool, element #5=w146:bool, element #6=w143:bool, element #7=→"Relay State":bool, element #8=→"Switch State":bool)  [unwired: 8 in]
            n133 = call <vilib>:"WSS.Generate.Digital.vi"("LF Wheel Speed Sensor Settings"="Front Driver WS.Settings") -> ("Bit1"=w202:bool, "Bit0"=w203:bool)  [unwired: 9 in]
            n134 = call <vilib>:"WSS.Generate.Digital.vi"("LF Wheel Speed Sensor Settings"="Front Passenger WS.Settings") -> ("Bit1"=w199:bool, "Bit0"=w200:bool)  [unwired: 9 in]
            n135 = call <vilib>:"WSS.Generate.Digital.vi"("LF Wheel Speed Sensor Settings"="Read Passenger WS.Settings") -> ("Bit1"=w196:bool, "Bit0"=w197:bool)  [unwired: 9 in]
            n136 = call <vilib>:"WSS.Generate.Digital.vi"("LF Wheel Speed Sensor Settings"="Rear Driver WS.Settings") -> ("Bit1"=w193:bool, "Bit0"=w194:bool)  [unwired: 9 in]
            n137 = call <vilib>:"PWM.Measure.Digital.vi"("State"=w146, "Settings"="PWM IN 1.Settings") -> ("Measurement"=→"PWM IN 1.Measure":T1)  [unwired: 8 in, 1 out]
            n138 = call <vilib>:"PWM.Measure.Digital.vi"("State"=w143, "Settings"="PWM IN 2.Settings") -> ("Measurement"=→"PWM IN 2.Measure":T1)  [unwired: 8 in, 1 out]
            n139 = call-poly <vilib>:"Measure Events.vi"("settings.<user name>"="settings.Cyl Inj 1", "register bus"=w226, "event"=w183) -> ("measured data"=w180:T41, "status.<user name>"=→"status.Cyl Inj 1":T4)  [unwired: 7 in]
            n140 = call-poly <vilib>:"Measure Events.vi"("settings.<user name>"="settings.Cyl Inj 2", "register bus"=w226, "event"=w171) -> ("measured data"=w168:T41, "status.<user name>"=→"status.Cyl Inj 2":T4)  [unwired: 7 in]
            n141 = call-poly <vilib>:"Measure Events.vi"("settings.<user name>"="settings.Cyl Inj 3", "register bus"=w226, "event"=w159) -> ("measured data"=w156:T41, "status.<user name>"=→"status.Cyl Inj 3":T4)  [unwired: 7 in]
            n142 = Build Array(w214, w213, w212, w211, "Key", w209, w208, "Switch") -> (w205:bool[])
            "Mod3.Monitor" <- w205
            n143 = Build Array(w203, w202) -> (w192:bool[])
            n144 = Build Array(w200, w199) -> (w191:bool[])
            n145 = Build Array(w197, w196) -> (w190:bool[])
            n146 = Build Array(w194, w193) -> (w189:bool[])
            n147 = call <vilib>:"Capture Event.vi"("event # to capture"=T32 1, "measured data"=w180) -> ("capture.<user name>"=→"capture.Cyl Inj 1.Event 1":T3)  [unwired: 9 in]
            n148 = call <vilib>:"Capture Event.vi"("event # to capture"=T32 2, "measured data"=w180) -> ("capture.<user name>"=→"capture.Cyl Inj 1.Event 2":T3)  [unwired: 9 in]
            n149 = call <vilib>:"Capture Event.vi"("event # to capture"=T32 3, "measured data"=w180) -> ("capture.<user name>"=→"capture.Cyl Inj 1.Event 3":T3)  [unwired: 9 in]
            n150 = call <vilib>:"Capture Event.vi"("event # to capture"=T32 4, "measured data"=w180) -> ("capture.<user name>"=→"capture.Cyl Inj 1.Event 4":T3)  [unwired: 9 in]
            n151 = call <vilib>:"Capture Event.vi"("event # to capture"=T32 1, "measured data"=w168) -> ("capture.<user name>"=→"capture.Cyl Inj 2.Event 1":T3)  [unwired: 9 in]
            n152 = call <vilib>:"Capture Event.vi"("event # to capture"=T32 2, "measured data"=w168) -> ("capture.<user name>"=→"capture.Cyl Inj 2.Event 2":T3)  [unwired: 9 in]
            n153 = call <vilib>:"Capture Event.vi"("event # to capture"=T32 3, "measured data"=w168) -> ("capture.<user name>"=→"capture.Cyl Inj 2.Event 3":T3)  [unwired: 9 in]
            n154 = call <vilib>:"Capture Event.vi"("event # to capture"=T32 4, "measured data"=w168) -> ("capture.<user name>"=→"capture.Cyl Inj 2.Event 4":T3)  [unwired: 9 in]
            n155 = call <vilib>:"Capture Event.vi"("event # to capture"=T32 1, "measured data"=w156) -> ("capture.<user name>"=→"capture.Cyl Inj 3.Event 1":T3)  [unwired: 9 in]
            n156 = call <vilib>:"Capture Event.vi"("event # to capture"=T32 2, "measured data"=w156) -> ("capture.<user name>"=→"capture.Cyl Inj 3.Event 2":T3)  [unwired: 9 in]
            n157 = call <vilib>:"Capture Event.vi"("event # to capture"=T32 3, "measured data"=w156) -> ("capture.<user name>"=→"capture.Cyl Inj 3.Event 3":T3)  [unwired: 9 in]
            n158 = call <vilib>:"Capture Event.vi"("event # to capture"=T32 4, "measured data"=w156) -> ("capture.<user name>"=→"capture.Cyl Inj 3.Event 4":T3)  [unwired: 9 in]
            n159 = Build Array (concatenate)(w192, w191, w190, w189) -> (w187:bool[])
            "Mod5.Monitor" <- w187
            n160 = call "Digital_Output_8Channels.vi"("States"=w205, "IO"=T34 {"DO 0"="Mod3/DIO7", "DO 1"="Mod3/DIO6", "DO 2"="Mod3/DIO3", "DO 3"="Mod3/DIO2", "DO 4"="Mod3/DIO4", "DO 5"="Mod3/DIO0", "DO 6"="Mod3/DIO1", "DO 7"="Mod3/DIO5"}) -> ()  [unwired: 1 in]
            n161 = call "Digital_Output_8Channels.vi"("States"=w187, "IO"=T34 {"DO 0"="Mod5/DIO0", "DO 1"="Mod5/DIO1", "DO 2"="Mod5/DIO2", "DO 3"="Mod5/DIO3", "DO 4"="Mod5/DIO6", "DO 5"="Mod5/DIO7", "DO 6"="Mod5/DIO4", "DO 7"="Mod5/DIO5"}) -> ()  [unwired: 1 in]
          }
        }
      }
      n162 = node-c288 ("Output Node")(w123) -> ()
      n163 = node-c288 ("Output Node")(w125) -> ()
    }
  }
